vi "tb_interleave two fft dit_host.vi"() -> ()   [LabVIEW 2011]
uses:
  <vilib>/Analysis/NI_AALPro.lvlib
  <vilib>/Analysis/2dsp.llb/Real FFT.vi
  <vilib>/Analysis/NI_AALBase.lvlib
panel:
  out "Log Error":dbl[](graph)
  out "Error":dbl[](graph)
  out "LabVIEW FLP DIT":dbl[](graph)
  out "size(s)":i32
  out "LabVIEW FLP":dbl[](graph)
  out "FXP Coregen":dbl[](graph)
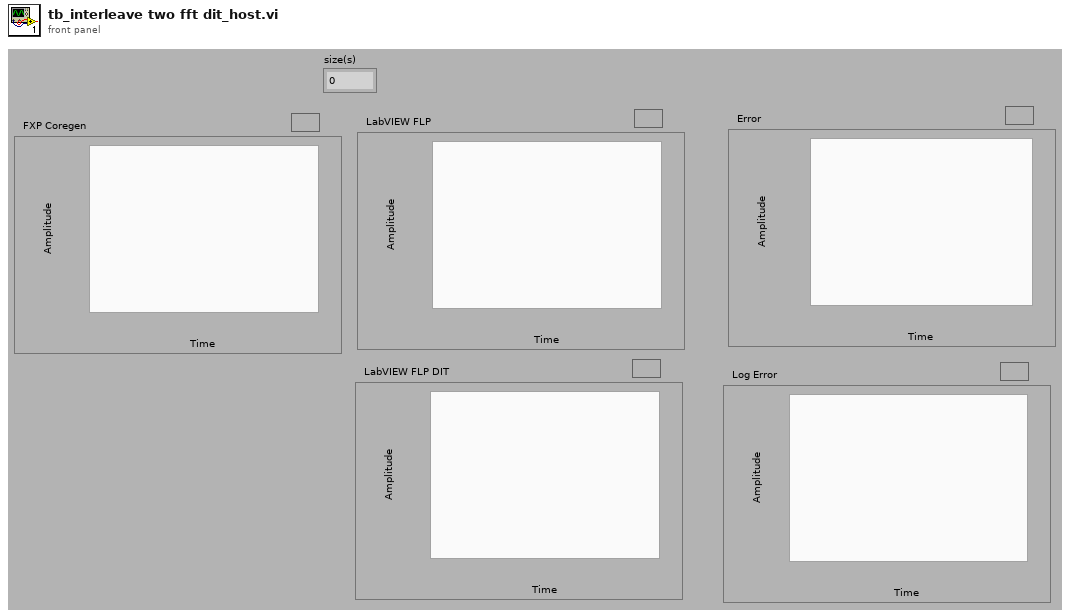
[diagram p1: front panel]
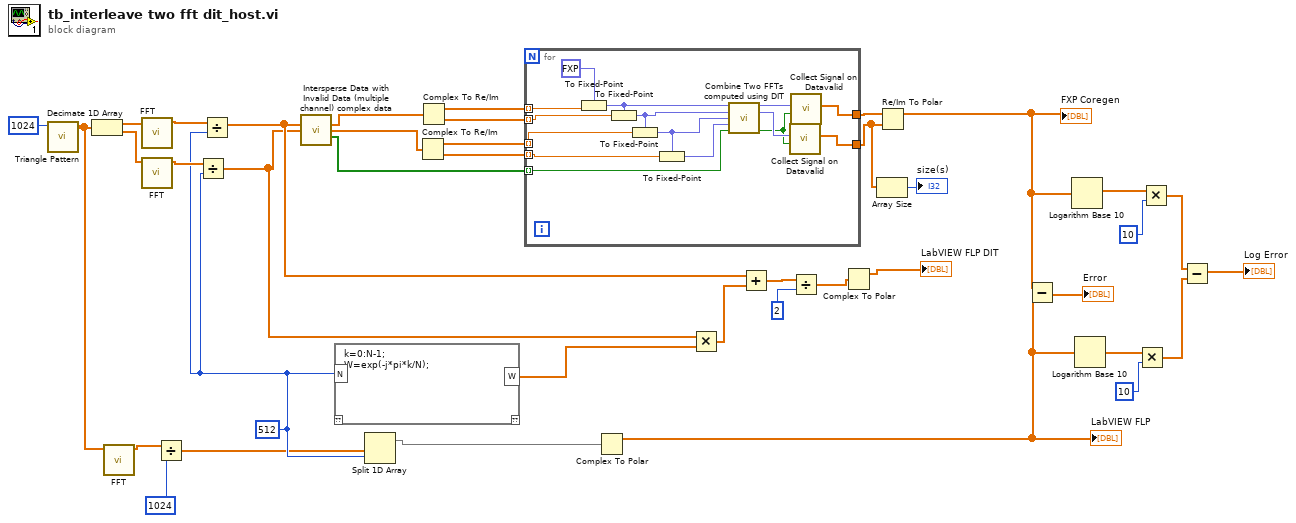
[diagram p0: block diagram]
diagram:
  w22 = 512 ("index")
  n1 = call <vilib>:"Triangle Pattern.vi"("samples"=1024) -> ("Triangle Pattern"=w32:dbl[])  [unwired: 9 in, 1 out]
  n2 = Decimate 1D Array(w32) -> (w34:dbl[], w33:dbl[])
  n3 = call-poly <vilib>:"FFT.vi"("X"=w32) -> ("FFT {X}"=w21:cdb[])  [unwired: 9 in, 1 out]
  n4 = call-poly <vilib>:"FFT.vi"("X"=w34) -> ("FFT {X}"=w24:cdb[])  [unwired: 9 in, 1 out]
  n5 = call-poly <vilib>:"FFT.vi"("X"=w33) -> ("FFT {X}"=w23:cdb[])  [unwired: 9 in, 1 out]
  n6 = Divide(x=w21, y=1024) -> (x/y=w19:cdb[])
  n7 = Divide(x=w23, y=w22) -> (x/y=w11:cdb[])
  n8 = Divide(x=w24, y=w22) -> (x/y=w12:cdb[])
  n9 = call <userlib>:"Intersperse Data with Invalid Data (multiple channel) complex data.vi"("Channel0 Input"=w12, "Channel1 Input"=w11) -> ("Channel0 Output"=w15:cdb[], "Channel1 Output"=w14:cdb[], "Data Valid"=w13:bool[])  [unwired: 11 in]
  n10 = mathscript code="k=0:N-1;\nW=exp(-j*pi*k/N);"("N"=w22) -> ("W"=w26:cdb[])  [unwired: 1 in, 1 out]
  n11 = Split 1D Array(array=w19, index=w22) -> (first subarray=w30:cdb[])  [unwired: 1 out]
  n12 = Complex To Re/Im(x + iy=w14) -> (x=w36:dbl[], y=w35:dbl[])
  n13 = Complex To Re/Im(x + iy=w15) -> (x=w38:dbl[], y=w37:dbl[])
  n14 = for {
    tunnel: w38 -> [w53] mode=indexing
    tunnel: w37 -> [w52] mode=indexing
    tunnel: w36 -> [w49] mode=indexing
    tunnel: w35 -> [w47] mode=indexing
    tunnel: [w43] -> w31
    tunnel: [w42] -> w29
    tunnel: w13 -> [w40] mode=indexing
    n15 = To Fixed-Point(fixed-point type=fxp<+/-,18,1> 0.0 ("Real FFT 1"), number=w53) -> (fixed-point=w51:fxp<+/-,18,1>)
    n16 = To Fixed-Point(fixed-point type=w51, number=w52) -> (fixed-point=w50:fxp<+/-,18,1>)
    n17 = To Fixed-Point(fixed-point type=w50, number=w49) -> (fixed-point=w48:fxp<+/-,18,1>)
    n18 = To Fixed-Point(fixed-point type=w48, number=w47) -> (fixed-point=w46:fxp<+/-,18,1>)
    n19 = call "Combine Two FFTs computed using DIT.vi"("Real FFT 1"=w51, "Imag FFT 1"=w50, "Real FFT 2"=w48, "Imag FFT 2"=w46, "Input Data Valid"=w40) -> ("Real FFT k"=w45:fxp<+/-,24,3>, "Imag FFT k"=w44:fxp<+/-,24,3>, "Output Valid"=w41:bool)  [unwired: 6 in, 2 out]
    n20 = call <userlib>:"Collect Signal on Datavalid.vi"("Data Valid"=w41, "Input"=w44) -> ("Output"=w42:dbl[])  [unwired: 9 in]
    n21 = call <userlib>:"Collect Signal on Datavalid.vi"("Data Valid"=w41, "Input"=w45) -> ("Output"=w43:dbl[])  [unwired: 9 in]
  }
  n22 = Complex To Polar(r * e^(i*theta)=w30) -> (r=w8:dbl[])  [unwired: 1 out]
  "LabVIEW FLP" <- w8
  n23 = Multiply(x=w11, y=w26) -> (x*y=w27:cdb[])
  n24 = Add(x=w12, y=w27) -> (x+y=w18:cdb[])
  n25 = Divide(x=w18, y=2 ("index")) -> (x/y=w16:cdb[])
  n26 = Complex To Polar(r * e^(i*theta)=w16) -> (r=→"LabVIEW FLP DIT":dbl[])  [unwired: 1 out]
  n27 = Array Size(array=w29) -> (size(s)=→"size(s)":i32)
  n28 = Re/Im To Polar(2:w29, 3:w31) -> (1:w9:dbl[])  [unwired: 1 out]
  "FXP Coregen" <- w9
  n29 = Subtract(x=w9, y=w8) -> (x-y=→"Error":dbl[])
  n30 = Logarithm Base 10(1:w9) -> (0:w7:dbl[])
  n31 = Logarithm Base 10(1:w8) -> (0:w4:dbl[])
  n32 = Multiply(x=w4, y=10) -> (x*y=w2:dbl[])
  n33 = Multiply(x=w7, y=10) -> (x*y=w3:dbl[])
  n34 = Subtract(x=w3, y=w2) -> (x-y=→"Log Error":dbl[])
